vi "Measurement Logic.vi"() -> ()   [LabVIEW 2024, in "NIDCPowerPPS.lvlib"]
uses:
  NIDCPowerPPS.lvlib
  Measurement Configuration.ctl
  Measurement Results.ctl
  <vilib>/MeasurementLink/MeasurementLink Measurement Server/Measure Call Context/Measure Call Context.lvclass
  <vilib>/MeasurementLink/MeasurementLink Measurement Server/Measure Call Context/Reserve Sessions - 1Pin.vi
  <vilib>/MeasurementLink/MeasurementLink niDCPower/Get Connections - 1Pin 1Conn.vi
  <vilib>/MeasurementLink/MeasurementLink niDCPower/Initialize Sessions - 1Sess.vi
  <vilib>/MeasurementLink/MeasurementLink niDCPower/MeasurementLink niDCPower.lvlib
  <vilib>/MeasurementLink/MeasurementLink Session Management V1/Session Reservation/Session Reservation.lvclass
panel:
  out "measure call context out":refnum<class "Measure Call Context.lvclass">
  in  "measure call context in":refnum<class "Measure Call Context.lvclass">
  out "measurement results":T1
  in  "measurement configuration":T2={"Pin Name"="Pin1", "Voltage Level (V)"=2.0, "Voltage Level Range (V)"=6.0, "Current Limit (A)"=0.01, "Current Limit Range (A)"=0.01, "Source Delay (s)"=0.1} {"Source Delay (s)" format="%#_6p"; "Current Limit Range (A)" format="%#_6p"; "Current Limit (A)" format="%#_6p"; "Voltage Level Range (V)" format="%#_6p"; "Voltage Level (V)" format="%#_6p"}
  out "error out":errorcluster
  in  "error in":errorcluster
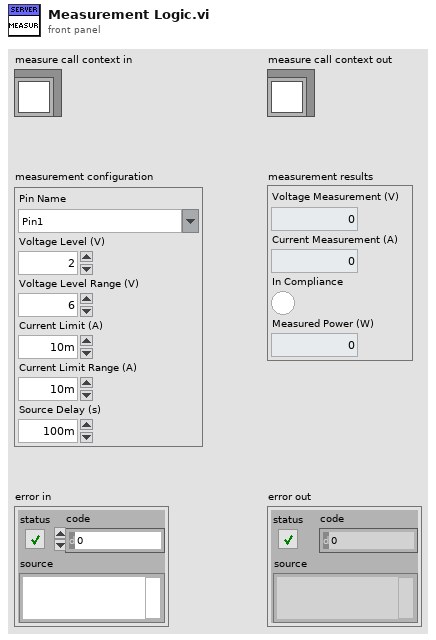
[diagram p1: front panel]
types:
  T1 = typedef "NIDCPowerPPS.lvlib/Measurement Results.ctl" = cluster{"Voltage Measurement (V)":dbl, "Current Measurement (A)":dbl, "In Compliance":bool, "Measured Power (W)":dbl}
  T2 = typedef "NIDCPowerPPS.lvlib/Measurement Configuration.ctl" = cluster{"Pin Name":string, "Voltage Level (V)":dbl, "Voltage Level Range (V)":dbl, "Current Limit (A)":dbl, "Current Limit Range (A)":dbl, "Source Delay (s)":dbl}
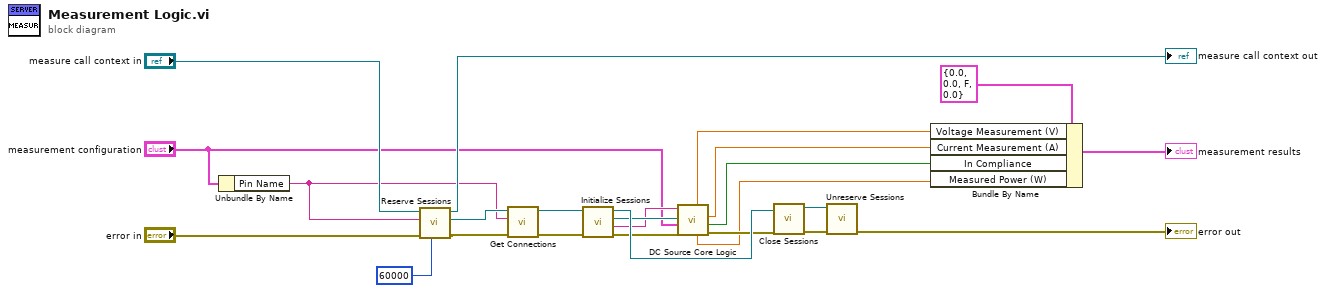
[diagram p0: block diagram]
diagram:
  n1 = Unbundle By Name("measurement configuration") -> ("Pin Name"=w7:string)
  n2 = call-poly <vilib>:"Reserve Sessions.vi"("timeout (ms)"=60000, "error in"="error in", "pin or relay name"=w7, "measurement context in"="measure call context in") -> ("error out"=w20:errorcluster, "session reservation out"=w18:refnum<class "Session Reservation.lvclass">, "measurement context out"=→"measure call context out":refnum<class "Measure Call Context.lvclass">)  [unwired: 5 in]
  n3 = call-poly <vilib>:"Get Connections.vi"("error in"=w20, "pin or relay name"=w7, "session reservation in"=w18) -> ("error out"=w22:errorcluster, "session reservation out"=w21:refnum<class "Session Reservation.lvclass">)  [unwired: 6 in, 1 out]
  n4 = call-poly <vilib>:"Initialize Sessions.vi"("error in"=w22, "session reservation in"=w21) -> ("error out"=w12:errorcluster, "channel list"=w13:string, "session"=w14:refnum<k15>, "session reservation out"=w15:refnum<class "Session Reservation.lvclass">)  [unwired: 6 in]
  n5 = call "DC Source Core Logic.vi"("error in"=w12, "measurement configuration"="measurement configuration", "instrument handle"=w14, "channel list"=w13) -> ("error out"=w11:errorcluster, "in compliance?"=w3:bool, "measured current"=w4:dbl, "calculated power"=w2:dbl, "measured voltage"=w5:dbl)  [unwired: 2 in, 1 out]
  n6 = call <vilib>:"Close Sessions.vi"("error in"=w11, "session reservation in"=w15) -> ("error out"=w17:errorcluster, "session reservation out"=w16:refnum<class "Session Reservation.lvclass">)  [unwired: 8 in]
  n7 = call <vilib>:"Unreserve Sessions.vi"("error in"=w17, "session reservation in"=w16) -> ("error out"=→"error out":errorcluster)  [unwired: 9 in]
  n8 = Bundle By Name(cluster=T1 {"Voltage Measurement (V)"=0.0, "Current Measurement (A)"=0.0, "In Compliance"=FALSE, "Measured Power (W)"=0.0} ("Measurement Results"), "Voltage Measurement (V)"=w5, "Current Measurement (A)"=w4, "In Compliance"=w3, "Measured Power (W)"=w2) -> (→"measurement results":T1)
